vi "dump.vi"(8 "error in (no error)":errorcluster, 10 "indent":T1, 11 "SsaId in":refnum<class "SsaId.lvclass">) -> (0 "error out":errorcluster, 2 "mlir":string, 3 "SsaId out":refnum<class "SsaId.lvclass">)   [LabVIEW 2020, in "mlir.lvlib" / "SsaId.lvclass"]
uses:
  SsaId.lvclass
  Node/indent.ctl
  SsaId.lvclass/SsaId.ctl
  Identifier/Identifier.lvclass
  mlir.lvlib
panel:
  # "Dumps the AST node and its children in MLIR format."
  # "String representing the AST in MLIR."
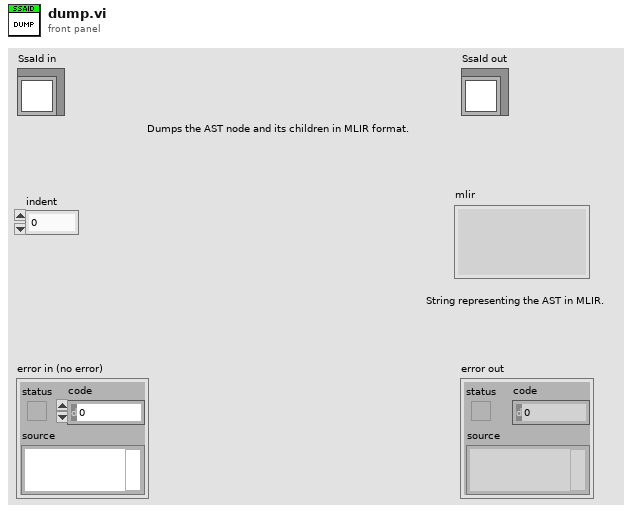
[diagram p1: front panel]
types:
  T1 = typedef "mlir.lvlib/indent.ctl" = u32
  T2 = typedef "mlir.lvlib/SsaId.lvclass/op_no.ctl" = u32
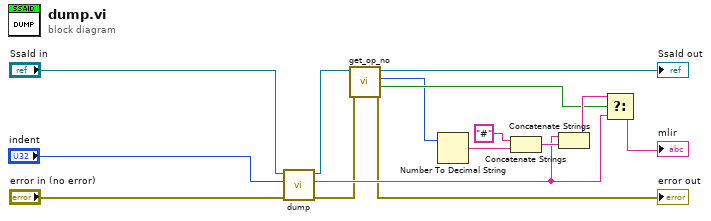
[diagram p0: block diagram]
diagram:
  n1 = call-parent "dump.vi"("error in (no error)"="error in (no error)", "indent"="indent", "self in"="SsaId in") -> ("error out"=w2:errorcluster, "mlir"=w8:string, "self out"=w6:refnum<class "SsaId.lvclass">)  [unwired: 6 in]
  n2 = call-dynamic "get_op_no.vi"("error in (no error)"=w2, "SsaId in"=w6) -> ("error out"=→"error out":errorcluster, "is_set?"=w4:bool, "op_no"=w3:T2, "SsaId out"=→"SsaId out":refnum<class "SsaId.lvclass">)  [unwired: 6 in]
  n3 = Number To Decimal String(number=w3) -> (decimal integer string=w11:string)  [unwired: 1 in]
  n4 = Concatenate Strings("#" ("string"), w11) -> (w10:string)
  n5 = Concatenate Strings(w8, w10) -> (w9:string)
  n6 = Select(t=w9, s=w4, f=w8) -> (s? t:f=→"mlir":string)
